vi "Mouse Move.vi"(8 "error in (no error)":errorcluster, 9 "Vertical":i32, 10 "Horizontal":i32, 11 "ColorSelector in":refnum<class "ColorSelector.lvclass">) -> (0 "error out":errorcluster, 3 "ColorSelector out":refnum<class "ColorSelector.lvclass">)   [LabVIEW 2015, in "ColorSelector.lvclass"]
doc: "This VI executes when the Mouse Move Event is sent back to the Event Handler due to the event in the Mouse Capture.vi. It converts the screen coordinates into the panel coordinates of the panel owning the QControl and then calls the methods to select the Grey or Color.\n<b> </b> <b> </b>\n©2017 Q Software Innovations, LLC (QSI)\nwritten by Quentin Alldredge\nproduced in LabVIEW 2015\n\nsupport@qsoftwareinnovations.com\nwww.qsoftwareinnovations.com\n\nAll rights reserved.\n\nRedistribution and use in source and binary forms, with or without modification, are permitted provided that the following conditions are met:\n\n * Redistributions of source code must retain the above copyright notice, this list of conditions and the following disclaimer.\n * Redistributions in binary form must reproduce the above copyright notice, this list of conditions and the following disclaimer in the documentation and/or other materials provided with the distribution.\n * Neither the name of Q Software Innovations, LLC. nor the names of its contributors may be used to endorse or promote products derived from this software without specific prior written permission.\n\nTHIS SOFTWARE IS PROVIDED BY THE COPYRIGHT HOLDERS AND CONTRIBUTORS \"AS IS\" AND ANY EXPRESS OR IMPLIED WARRANTIES, INCLUDING, BUT NOT LIMITED TO, THE IMPLIED WARRANTIES OF MERCHANTABILITY AND FITNESS FOR A PARTICULAR PURPOSE ARE DISCLAIMED. IN NO EVENT SHALL THE COPYRIGHT OWNER OR CONTRIBUTORS BE LIABLE FOR ANY DIRECT, INDIRECT, INCIDENTAL, SPECIAL, EXEMPLARY, OR CONSEQUENTIAL DAMAGES (INCLUDING, BUT NOT LIMITED TO, PROCUREMENT OF SUBSTITUTE GOODS OR SERVICES; LOSS OF USE, DATA, OR PROFITS; OR BUSINESS INTERRUPTION) HOWEVER CAUSED AND ON ANY THEORY OF LIABILITY, WHETHER IN CONTRACT, STRICT LIABILITY, OR TORT (INCLUDING NEGLIGENCE OR OTHERWISE) ARISING IN ANY WAY OUT OF THE USE OF THIS SOFTWARE, EVEN IF ADVISED OF THE POSSIBILITY OF SUCH DAMAGE."
uses:
  ColorSelector.lvclass
  <vilib>/Utility/miscctls.llb/LVPoint32TypeDef.ctl
  ColorSelector.lvclass/ColorSelector.ctl
  Read ActiveSelector.vi
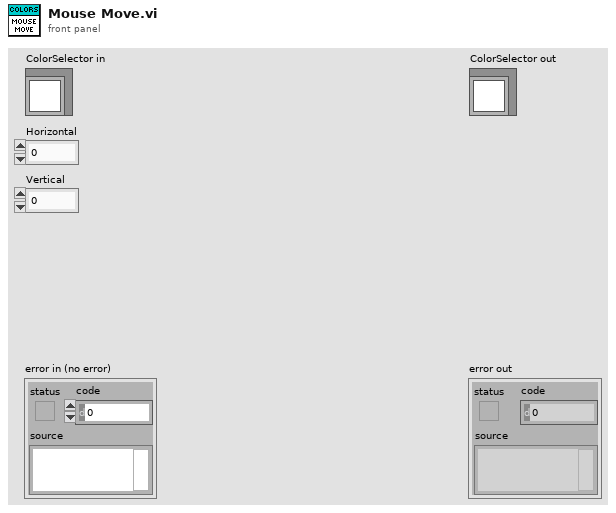
[diagram p1: front panel]
types:
  T1 = typedef "LVPoint32TypeDef.ctl" = cluster{"Horizontal":i32, "Vertical":i32}
  T2 = typedef "LVRectTypeDef.ctl" = cluster{"Left":i16, "Top":i16, "Right":i16, "Bottom":i16}
  T3 = typedef "ColorSelector.lvclass/Active Selector Enum.ctl" = enum16{"Grey", "Color"}
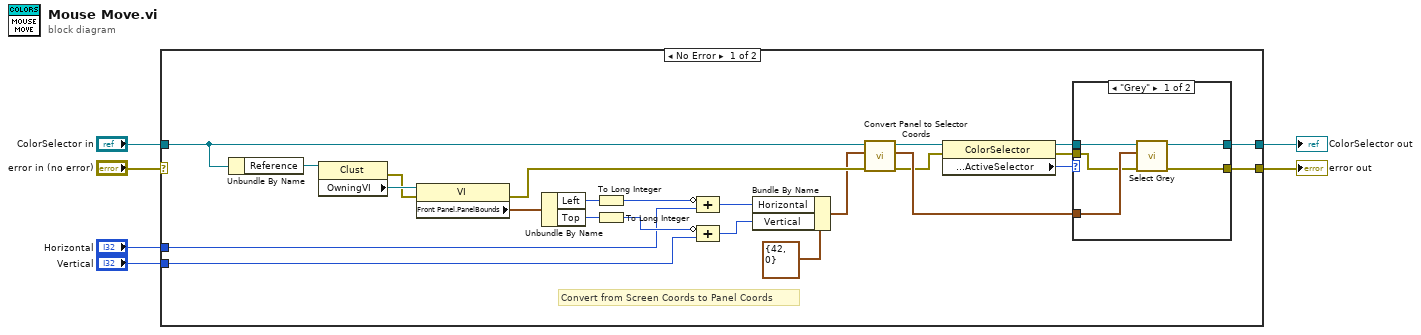
[diagram p0: block diagram]
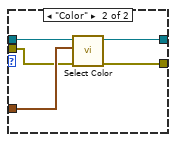
[diagram p2: hidden frame]
diagram:
  n1 = case shown="No Error" "error in (no error)" {
    selector: "error in (no error)" -> [_ w42]
    tunnel: [w21 w42] -> w5
    tunnel: [w23 w41] -> w3
    tunnel: "ColorSelector in" -> [w8 w41]
    tunnel: "Horizontal" -> [w14 _]
    tunnel: "Vertical" -> [w13 _]
    frame No Error {
      # "Convert from Screen Coords to Panel Coords"
      n2 = Unbundle By Name(w8) -> ("Reference"=w29:refnum<vi>)
      n3 = property class="Clust"(reference=w29) -> (error out=w22:errorcluster, "OwningVI"=w30:refnum<vi>)  [unwired: 1 in, 1 out]
      n4 = property class="VI"(reference=w30, error in=w22) -> (error out=w12:errorcluster, "Front Panel.PanelBounds"=w28:T2)  [unwired: 1 out]
      n5 = Unbundle By Name(w28) -> ("Left"=w27:i16, "Top"=w26:i16)
      n6 = To Long Integer(number=w27) -> (32bit integer=w16:i32)
      n7 = To Long Integer(number=w26) -> (32bit integer=w15:i32)
      n8 = Compound Arithmetic op=ADD(invert w16, w14) -> (w25:i32)
      n9 = Compound Arithmetic op=ADD(invert w15, w13) -> (w24:i32)
      n10 = Bundle By Name(cluster=T1 {"Horizontal"=42, "Vertical"=0} ("Coords"), "Horizontal"=w25, "Vertical"=w24) -> (w11:T1)
      n11 = call "Convert Panel to Selector Coords.vi"("error in (no error)"=w12, "Coords in (Panel)"=w11, "ColorSelector in"=w8) -> ("error out"=w9:errorcluster, "Coords in (Control)"=w10:T1, "ColorSelector (dup)"=w7:refnum<class "ColorSelector.lvclass">)  [unwired: 6 in]
      n12 = property class="ColorSelector"(reference=w7, error in=w9) -> (reference out=w19:refnum<class "ColorSelector.lvclass">, error out=w18:errorcluster, "State Data:Accessors:ActiveSelector"=w20:T3)
      n13 = case shown="\"Grey\"" w20 {
        tunnel: w10 -> [w32 w37]
        tunnel: [w35 w39] -> w23
        tunnel: w18 -> [w31 w36]
        tunnel: [w34 w40] -> w21
        tunnel: w19 -> [w33 w38]
        frame "Grey" {
          n14 = call "Select Grey.vi"("error in (no error)"=w31, "Coords"=w32, "ColorSelector in"=w33) -> ("error out"=w34:errorcluster, "ColorSelector out"=w35:refnum<class "ColorSelector.lvclass">)  [unwired: 7 in]
        }
        frame "Color" {
          n15 = call "Select Color.vi"("error in (no error)"=w36, "Coords in"=w37, "ColorSelector in"=w38) -> ("error out"=w40:errorcluster, "ColorSelector (dup)"=w39:refnum<class "ColorSelector.lvclass">)  [unwired: 7 in]
        }
      }
    }
    frame Error {
    }
  }
  "error out" <- w5
  "ColorSelector out" <- w3
